vi "SMU Config - PAE.vi"(7 "Test Configuration":T1={"Expected DUT Gain (dB)"=17.5, "Max Linear Range (dBm)"=-10.0, "Compression Point (dB)"=1.0, "Pout at Pin (dBm)"=1.0, "RFSG Frequency Start (Hz)"=6000000000.0, "RFSG Frequency Stop (Hz)"=18000000000.0, "RFSG Number of Frequency Step"=10, "Power Start (dBm)"=-20.0, "Power Stop(dBm)"=1.0, "Power Step Size (dB)"=4.0, "RBW (Hz)"=5000000.0, "Modes"={"RF Measurement Interval (s)"=0.001, "DC Measurement Interval (s)"=0.0, "Power Stimulus Mode"=enum."Constant Power and RF", "CP_CW_DC Source Delay (s)"=0.0002, "CP_PRF_RF Pulse Width (s)"=0.0009, "CP_PRF_PRI (s)"=0.015, "CP_PRF_DC Source Delay (s)"=0.0, "CP_PRF_RFmx Trigger Delay (s)"=0.2, "PP_PRF_RF Pulse Width (s)"=0.0, "PP_PRF_PRI (s)"=0.0, "PP_PRF_DC Pulse Width (s)"=0.0008, "PP_PRF_Bias Voltage Level (V)"=0.0, "PP_PRF_Bias Current Limit (A)"=0.2, "PP_PRF_DC Source Delay (s)"=0.0, "PP_PRF_RFmx Trigger Delay (s)"=0.0}} {"Pout at Pin (dBm)" format="%#pdBm"; "Modes"."PP_PRF_RFmx Trigger Delay (s)" format="%#ps"; "Modes"."PP_PRF_DC Source Delay (s)" format="%#ps"; "Modes"."PP_PRF_Bias Current Limit (A)" format="%#pA"; "Modes"."PP_PRF_Bias Voltage Level (V)" format="%#pV"; "Modes"."PP_PRF_DC Pulse Width (s)" format="%#ps"; "Modes"."PP_PRF_PRI (s)" format="%#ps"; "Modes"."PP_PRF_RF Pulse Width (s)" format="%#ps"; "Modes"."CP_PRF_RFmx Trigger Delay (s)" format="%#ps"; "Modes"."CP_PRF_DC Source Delay (s)" format="%#ps"; "Modes"."CP_PRF_PRI (s)" format="%#ps"; "Modes"."CP_PRF_RF Pulse Width (s)" format="%#ps"; "Modes"."CP_CW_DC Source Delay (s)" format="%#ps"; "Modes"."DC Measurement Interval (s)" format="%#_6p"; "RFSG Frequency Stop (Hz)" format="%#_6p"; "Power Start (dBm)" format="%#_6p"; "Power Stop(dBm)" format="%#_6p"; "RFSG Frequency Start (Hz)" format="%#_6p"; "Expected DUT Gain (dB)" step=1.0 format="%#_6p"}, 8 "error in":errorcluster, 10 "SMU Settings":T3, 11 "Data Value Reference in":T2) -> (0 "error out":errorcluster, 2 "voltage measurements":dbl[](array[numeric]), 3 "Data Value Reference out":T2)   [LabVIEW 2023]
uses:
  Controls/SMU Config - Compression.ctl
  <vilib>/niPAEML/Typedefs/Session Handle.ctl
  <vilib>/niPAEML/PAE Reference.lvclass
  Controls/Test Config - Compression.ctl
  <instrlib>/niDCPower/nidcpower.llb/niDCPower gRPC Device Server.ctl
  <vilib>/niPAEML/PAE Measurement.lvlib
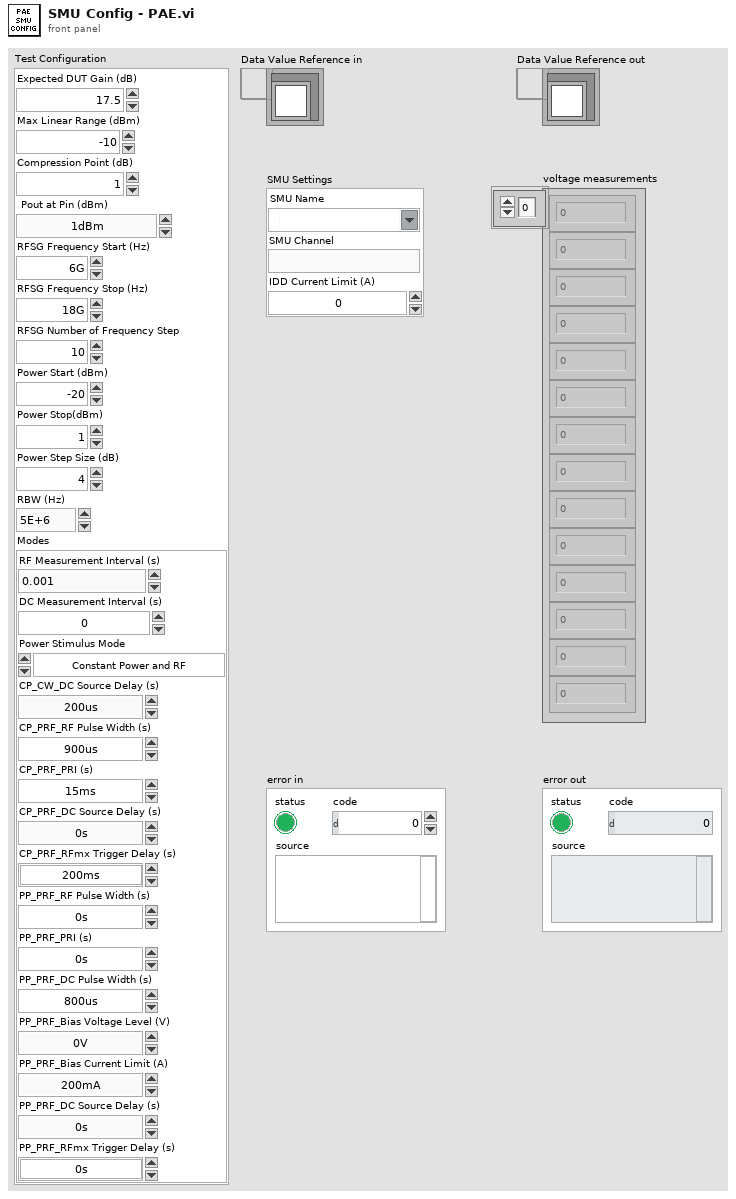
[diagram p1: front panel]
types:
  T1 = typedef "Test Config - Compression.ctl" = cluster{"Expected DUT Gain (dB)":dbl, "Max Linear Range (dBm)":dbl, "Compression Point (dB)":dbl, "Pout at Pin (dBm)":dbl, "RFSG Frequency Start (Hz)":dbl, "RFSG Frequency Stop (Hz)":dbl, "RFSG Number of Frequency Step":i32, "Power Start (dBm)":dbl, "Power Stop(dBm)":dbl, "Power Step Size (dB)":dbl, "RBW (Hz)":dbl, "Modes":cluster{"RF Measurement Interval (s)":dbl, "DC Measurement Interval (s)":dbl, "Power Stimulus Mode":enum16{"Constant Power and RF", "Constant Power and Pulsed RF", "Pulsed Power and RF"}, "CP_CW_DC Source Delay (s)":dbl, "CP_PRF_RF Pulse Width (s)":dbl, "CP_PRF_PRI (s)":dbl, "CP_PRF_DC Source Delay (s)":dbl, "CP_PRF_RFmx Trigger Delay (s)":dbl, "PP_PRF_RF Pulse Width (s)":dbl, "PP_PRF_PRI (s)":dbl, "PP_PRF_DC Pulse Width (s)":dbl, "PP_PRF_Bias Voltage Level (V)":dbl, "PP_PRF_Bias Current Limit (A)":dbl, "PP_PRF_DC Source Delay (s)":dbl, "PP_PRF_RFmx Trigger Delay (s)":dbl}}
  T2 = typedef "PAE Measurement.lvlib/PAE Reference.lvclass/Session Handle.ctl" = refnum<data-value>
  T3 = typedef "SMU Config - Compression.ctl" = cluster{"SMU Name":refnum<k15>, "SMU Channel":string, "IDD Current Limit (A)":dbl}
  T4 = typedef "niDCPower gRPC Device Server.ctl" = cluster{"session name":string, "address (localhost)":string, "port (31763)":u32}
  T5 = enum16{"Constant Power and RF", "Constant Power and Pulsed RF", "Pulsed Power and RF"}
  T6 = cluster{"Source Mode":i32, "Output Function":i32, "Output Enabled":bool, "Voltage Level":dbl, "Voltage Level Range":dbl, "Voltage Level Autorange":i32, "Current Limit":dbl, "Current Limit Range":dbl, "Current Limit Autorange":i32, "Source Delay":dbl, "Aperture Time":dbl, "Measure Record Length":i32, "Measure Record Length Is Finite":bool, "Measure When":i32, "Measure Trigger Type":i32, "Exported Measure Trigger Output Terminal":string, "Measure Trigger Digital Edge - Edge":i32, "Measure Trigger Digital Edge - Input Terminal":string, "Sequence Advance Trigger Type":i32, "Exported Sequence Advance Trigger Output Terminal":string, "Sequence Advance Trigger Digital Edge - Edge":i32, "Sequence Advance Trigger Digital Edge - Input Terminal":string}
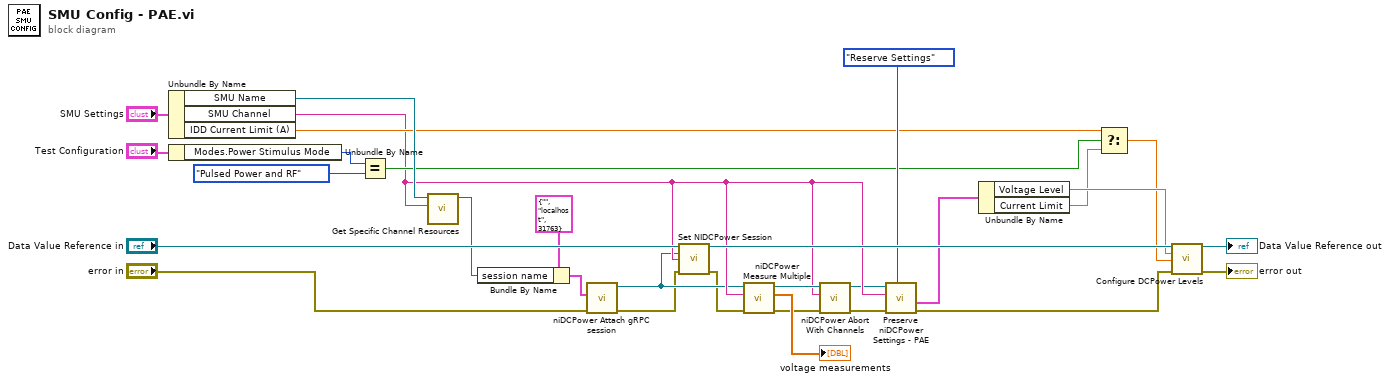
[diagram p0: block diagram]
diagram:
  n1 = Unbundle By Name("SMU Settings") -> ("SMU Name"=w30:refnum<k15>, "SMU Channel"=w5:string, "IDD Current Limit (A)"=w11:dbl)
  n2 = Unbundle By Name("Test Configuration") -> ("Modes.Power Stimulus Mode"=w14:T5)
  n3 = Equal?(x=w14, y=T5."Pulsed Power and RF") -> (x = y?=w12:bool)
  n4 = call "Get Specific Channel Resources.vi"("Channel"=w5, "Resource Name"=w30) -> ("Resource Name"=w7:refnum<k15>)  [unwired: 9 in]
  n5 = Bundle By Name(cluster=T4 {"session name"="", "address (localhost)"="localhost", "port (31763)"=31763} ("gRPC options"), "session name"=w7) -> (w9:T4)
  n6 = call <instrlib>:"niDCPower Attach gRPC session.vi"("error in (no error)"="error in", "gRPC options"=w9) -> ("error out"=w3:errorcluster, "instrument handle out"=w4:refnum<k15>)  [unwired: 8 in]
  n7 = call <vilib>:"Set NIDCPower Session.vi"("PAE Reference In"="Data Value Reference in", "NI DCPower Instrument Handle"=w4, "NI DCPower Channel Name"=w5, "error in"=w3) -> ("PAE Reference Out"=w23:T2, "error out"=w2:errorcluster)  [unwired: 10 in]
  n8 = call <instrlib>:"niDCPower Measure Multiple.vi"("error in (no error)"=w2, "channel name"=w5, "instrument handle"=w4) -> ("error out"=w27:errorcluster, "voltage measurements"=→"voltage measurements":dbl[], "instrument handle out"=w25:refnum<k15>)  [unwired: 5 in, 1 out]
  n9 = call <instrlib>:"niDCPower Abort With Channels.vi"("error in (no error)"=w27, "channel name"=w5, "instrument handle"=w25) -> ("error out"=w26:errorcluster, "instrument handle out"=w1:refnum<k15>)  [unwired: 7 in]
  n10 = call "Preserve niDCPower Settings - PAE.vi"("Action"=enum16{"Reserve Settings", "Re-apply Settings"}."Reserve Settings", "error in"=w26, "Active Channel"=w5, "Resource Name"=w1) -> ("error out"=w22:errorcluster, "output cluster"=w19:T6)  [unwired: 4 in, 2 out]
  n11 = Unbundle By Name(w19) -> ("Voltage Level"=w18:dbl, "Current Limit"=w10:dbl)
  n12 = Select(t=w11, s=w12, f=w10) -> (s? t:f=w16:dbl)
  n13 = call <vilib>:"Configure DCPower Levels.vi"("PAE Reference In"=w23, "Voltage Level (V)"=w18, "Current Limit (A)"=w16, "error in"=w22) -> ("PAE Reference Out"=→"Data Value Reference out":T2, "error out"=→"error out":errorcluster)  [unwired: 10 in]
